vi "C64_main_T.vi"() -> ()   [LabVIEW 2018]
uses:
  CPU/CPU_registers.ctl
panel:
  in  "reset":bool
  in  "stop":bool
  out "registers":T1 {"P" format="%08b"; "PC" format="%04x"; "SP" format="%02x"; "Y" format="%02x"; "X" format="%02x"; "A" format="%02x"}
  out "ticks/s":u32 format="%.2p"
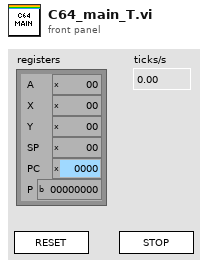
[diagram p1: front panel]
types:
  T1 = typedef "CPU_registers.ctl" = cluster{"A":u8, "X":u8, "Y":u8, "SP":u8, "PC":u16, "P":u8}
  T2 = enum32{"Invalid", "Standard", "Closed", "Hidden", "Minimized", "Maximized"}
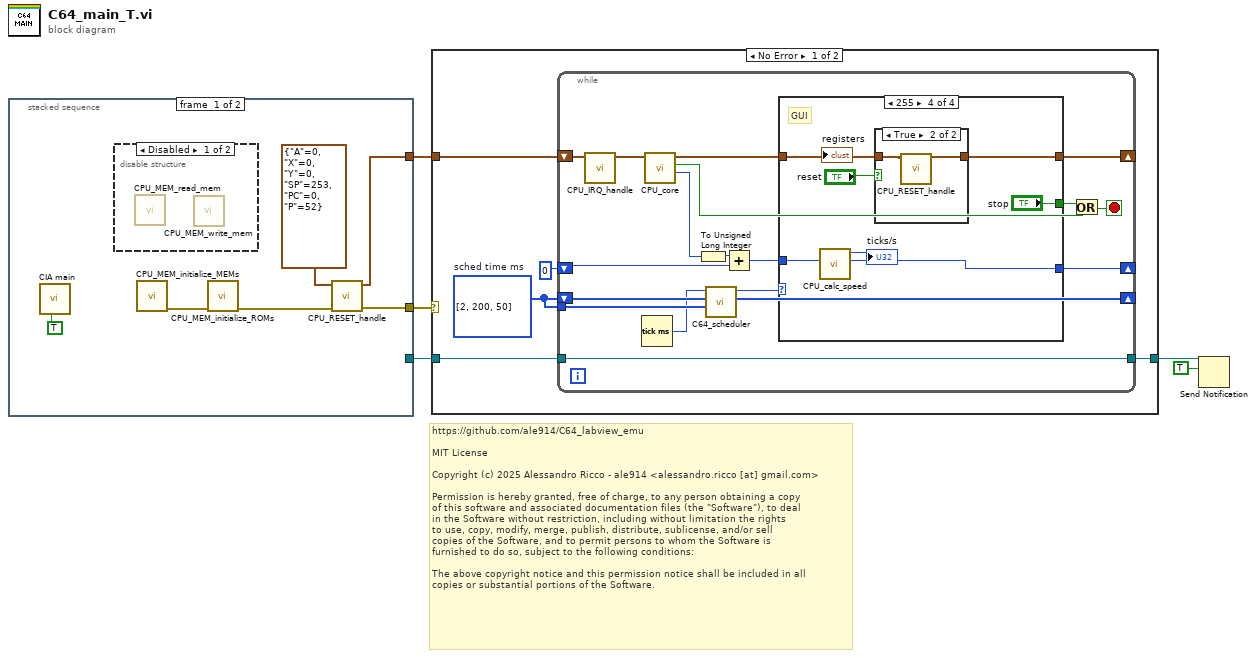
[diagram p0: block diagram]
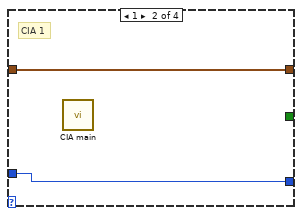
[diagram p3: hidden frame]
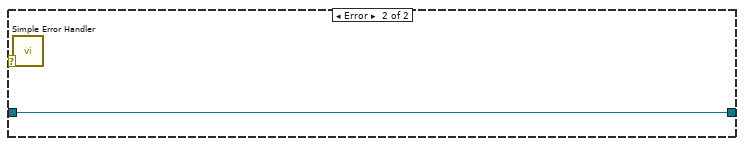
[diagram p6: hidden frame]
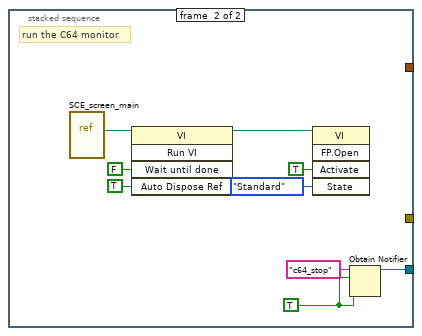
[diagram p8: hidden frame]
diagram:
  # "https://github.com/ale914/C64_labview_emu\n\nMIT License\n\nCopyright (c) 2025 Alessandro Ricco - ale914 <alessandro.ricco [at] gmail.com>\n\nPermission is hereby granted, free of charge, to any person obtaining a copy\nof this software and associated documentation files (the \"Software\"), to deal\nin the Software without restriction, including without limitation the rights\nto use, copy, modify, merge, publish, distribute, sublicense, and/or sell\ncopies of the Software, and to permit persons to whom the Software is\nfurnished to do so, subject to the following conditions:\n\nThe above copyright notice and this permission notice shall be included in all\ncopies or substantial portions of the Software."
  n1 = stacked-sequence {
    tunnel: [w8 _] -> w5
    tunnel: [_ w12] -> w4
    tunnel: [w6 _] -> w1
    frame #0 {
      n2 = call "CIA main.vi"("init"=TRUE) -> ()  [unwired: 11 in]
      n3 = disable-structure shown="Disabled" {
        frame Disabled {
          n4 = call "CPU_MEM_read_mem.vi"() -> ()  [unwired: 11 in, 1 out]
          n5 = call "CPU_MEM_write_mem.vi"() -> ()  [unwired: 12 in]
        }
        frame Enabled {
        }
      }
      n6 = call "CPU_MEM_initialize_MEMs.vi"() -> ("error out"=w10:errorcluster)  [unwired: 11 in]
      n7 = call "CPU_MEM_initialize_ROMs.vi"("error in (no error)"=w10) -> ("error out"=w7:errorcluster)  [unwired: 10 in]
      n8 = call "CPU_RESET_handle.vi"("error in (no error)"=w7, "registers"=T1 {"A"=0, "X"=0, "Y"=0, "SP"=253, "PC"=0, "P"=52} ("registers init")) -> ("error out"=w6:errorcluster, "registers"=w8:T1)  [unwired: 8 in]
    }
    frame #1 {
      w13 = TRUE ("create if not found? (T)")
      # "run the C64 monitor"
      n9 = vi-ref "SCE_screen_main.vi"() -> (w20:refnum<vi>)
      n10 = invoke class="VI" method="Run VI"(reference=w20, "Wait until done"=FALSE ("Wait Until Done"), "Auto Dispose Ref"=TRUE ("Auto Dispose Reference")) -> (reference out=w17:refnum<vi>)  [unwired: 2 in, 4 out]
      n11 = invoke class="VI" method="FP.Open"(reference=w17, "Activate"=TRUE ("Activate?"), "State"=T2."Standard") -> ()  [unwired: 2 in, 5 out]
      n12 = Obtain Notifier(name (unnamed)="c64_stop", notification data type=w13, create if not found? (T)=w13) -> (notifier out=w12:refnum<notifier>)  [unwired: 1 in, 2 out]
    }
  }
  n13 = case shown="No Error" w1 {
    selector: w1 -> [_ w60]
    tunnel: w5 -> [w23 _]
    tunnel: w4 -> [w22 w61]
    tunnel: [w21 w61] -> w3
    frame No Error {
      w24 = u32[] [2, 200, 50]  # sched time ms
      n14 = while {
        shift-right: [w37] -> _
        shift-left: w23 -> [w35]
        shift-right: [w39] -> _
        shift-left: w24 -> [w40]
        tunnel: w24 -> [w33]
        shift-right: [w28] -> _
        shift-left: u32 0 ("y") -> [w30]
        tunnel: w22 -> [w26]
        tunnel: [w26] -> w21
        stop <- w43 stop-if-true
        n15 = call "CPU_IRQ_handle.vi"("registers"=w35) -> ("registers"=w41:T1)  [unwired: 10 in]
        n16 = Tick Count (ms)() -> (millisecond timer value=w32:u32)
        n17 = call "CPU_core.vi"("registers"=w41) -> ("clock ticks"=w34:u8, "error"=w42:bool, "registers"=w27:T1)  [unwired: 8 in]
        n18 = To Unsigned Long Integer(number=w34) -> (unsigned 32bit integer=w31:u32)
        n19 = call "C64_scheduler.vi"("periods"=w33, "next time in"=w40, "global clock"=w32) -> ("next time out"=w39:u32[], "chip"=w38:u8)  [unwired: 7 in]
        n20 = Add(x=w31, y=w30) -> (x+y=w29:u32)
        n21 = case shown="255" w38 {
          tunnel: w27 -> [w45 w47 w49 w53]
          tunnel: [w45 w47 w49 w55] -> w37
          tunnel: [_ _ _ "stop"] -> w36
          tunnel: w29 -> [w44 w46 w48 w51]
          tunnel: [w44 w46 w48 w50] -> w28
          frame Default {
          }
          frame 1 {
            # "CIA 1"
            n22 = call "CIA main.vi"() -> ()  [unwired: 12 in]
          }
          frame 3 {
            # "VIC"
          }
          frame 255 {
            # "GUI"
            n23 = call "CPU_calc_speed.vi"("clock ticks"=w51) -> ("clock ticks out"=w50:u32, "ticks/s"=→"ticks/s":u32)  [unwired: 9 in]
            n24 = case shown="True" "reset" {
              tunnel: w53 -> [w57 w59]
              tunnel: [w57 w58] -> w55
              frame False {
              }
              frame True {
                n25 = call "CPU_RESET_handle.vi"("registers"=w59) -> ("registers"=w58:T1)  [unwired: 9 in, 1 out]
              }
            }
            "registers" <- w53
          }
        }
        n26 = Or(x=w36, y=w42) -> (x .or. y?=w43:bool)
      }
    }
    frame Error {
      n27 = call <vilib>:"Simple Error Handler.vi"("error in (no error)"=w60) -> ()  [unwired: 4 in, 5 out]
    }
  }
  n28 = Send Notification(notification=TRUE, notifier=w3) -> ()  [unwired: 1 in, 2 out]
